vi "Task_Detect_Calibration_Calculate_Tester_Parameter.vi"(11 "DDM Parameter":dbl[](array[numeric])) -> (3 "Calculate Tester Parameter":dbl[](array[numeric]))   [LabVIEW 2017]
panel:
  out "DDM Measured Power":dbl
  out "DDM Pressure":dbl
  out "DDM Speed":dbl
  out "DDM Power":dbl
  out "DDM Current":dbl
  out "DDM Voltage":dbl
  out "power":dbl
  out "current":dbl
  out "voltage":dbl
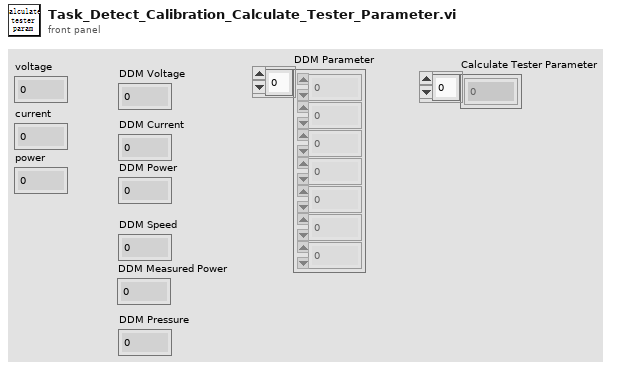
[diagram p1: front panel]
types:
  T1 = typedef "HD Config.ctl" = cluster{" PC":cluster{"PC Address":u8[], "PC Port":i32}, "FCO":cluster{"COM":refnum<visa-resource-name>, "Baudrate":u32}, "DC Power ":cluster{"COM":refnum<visa-resource-name>, "Baudrate":u32}, "PW3336":cluster{"COM":refnum<visa-resource-name>, "Baudrate":u32}, "Lefoo":cluster{"COM":refnum<visa-resource-name>, "Baudrate":u32}, "AI Model":cluster{"COM":refnum<visa-resource-name>, "Baudrate":u32}, "DIPC":cluster{"COM":refnum<visa-resource-name>}, "RFID":cluster{"IP Address":string, "Port":u16, "Retry":u16}, "Motor":cluster{"COM":refnum<visa-resource-name>, "Baudrate":u32}, "Fail_resume_mode":bool, "GRR":bool}
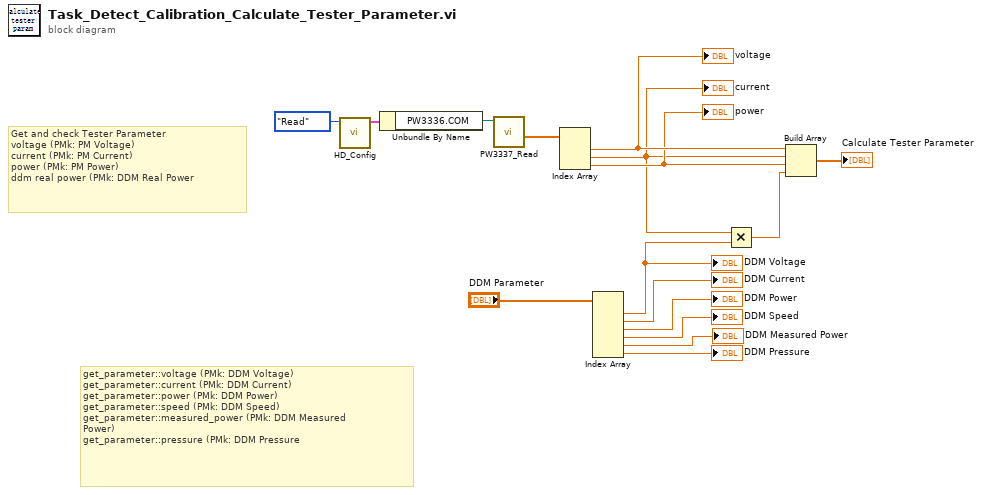
[diagram p0: block diagram]
diagram:
  # "Get and check Tester Parameter\nvoltage (PMk: PM Voltage)\ncurrent (PMk: PM Current)\npower (PMk: PM Power)\nddm real power (PMk: DDM Real Power"
  # "get_parameter::voltage (PMk: DDM Voltage)\nget_parameter::current (PMk: DDM Current)\nget_parameter::power (PMk: DDM Power)\nget_parameter::speed (PMk: DDM Speed)\nget_parameter::measured_power (PMk: DDM Measured \nPower)\nget_parameter::pressure (PMk: DDM Pressure"
  n1 = call "HD_Config.vi"("Step"=enum16{"Initial", "Write", "Read"}."Read") -> ("HD Config out"=w3:T1)  [unwired: 9 in, 1 out]
  n2 = Unbundle By Name(w3) -> ("PW3336.COM"=w2:refnum<visa-resource-name>)
  n3 = call "PW3337_Read.vi"("VISA resource name"=w2) -> ("Measurement out"=w1:dbl[])  [unwired: 7 in, 3 out]
  n4 = Index Array(array=w1) -> (element #1=w9:dbl, element #2=w6:dbl, element #3=w8:dbl)  [unwired: 3 in]
  "voltage" <- w9
  "current" <- w6
  "power" <- w8
  n5 = Index Array(array="DDM Parameter") -> (element #1=w7:dbl, element #2=→"DDM Current":dbl, element #3=→"DDM Power":dbl, element #4=→"DDM Speed":dbl, element #5=→"DDM Measured Power":dbl, element #6=→"DDM Pressure":dbl)  [unwired: 6 in]
  "DDM Voltage" <- w7
  n6 = Multiply(x=w6, y=w7) -> (x*y=w5:dbl)
  n7 = Build Array(w9, w6, w8, w5) -> (→"Calculate Tester Parameter":dbl[])
